vi "Autonomous Independent.vi"() -> ()   [LabVIEW 2020]
doc: "This VI is called when autonomous begins, and will automatically be terminated when autonomous ends. You can carry out timed or sensor driven robot movement independently without needing to return to the caller."
uses:
  <vilib>/Rock Robotics/WPI/Utilities/WPI_GetSetVariantRefNum.vi
  <vilib>/Rock Robotics/Network Tables/NT Read String.vi
  <vilib>/Rock Robotics/Network Tables/NT Write Numeric Array.vi
  <vilib>/Rock Robotics/Network Tables/NT Read Number.vi
  Robot Global Data.vi
  SUB VIs/TOGGLE GLOBAL.vi
  <vilib>/addons/control/pid/pid.llb/PID (DBL).vi
  ENUM_01.ctl
  <vilib>/addons/control/pid/NI_PID_pid.lvlib
panel:
  in  "CONTROL FREIO A3 2":dbl=-12.6
  in  "ACELERA敲O 3 A3 2":dbl=0.15
  in  "ACELERA敲O\n 3 A3 4":dbl=0.3
  in  "DISTANCE\nVOLTAR":dbl=1.6
  in  "TIMER 3 A3 2":dbl=500.0
  in  "ACELERA敲O 2 A3 2":dbl=-0.35
  in  "DISTANCIA A\nPERCORRER 2 A3 2":dbl=-4.0
  in  "TIMER 2 A3 2":dbl=50.0
  in  "DISTANCIA A\nPERCORRER 1 A3 2":dbl=0.1
  in  "ACELERA敲O 1 A3 2":dbl=0.3
  in  "TIMER 1 A3 2":dbl=150.0
  # "Be sure to right-click and choose Data Operations>>Make Current Value default if you want to save the array values with the VI"
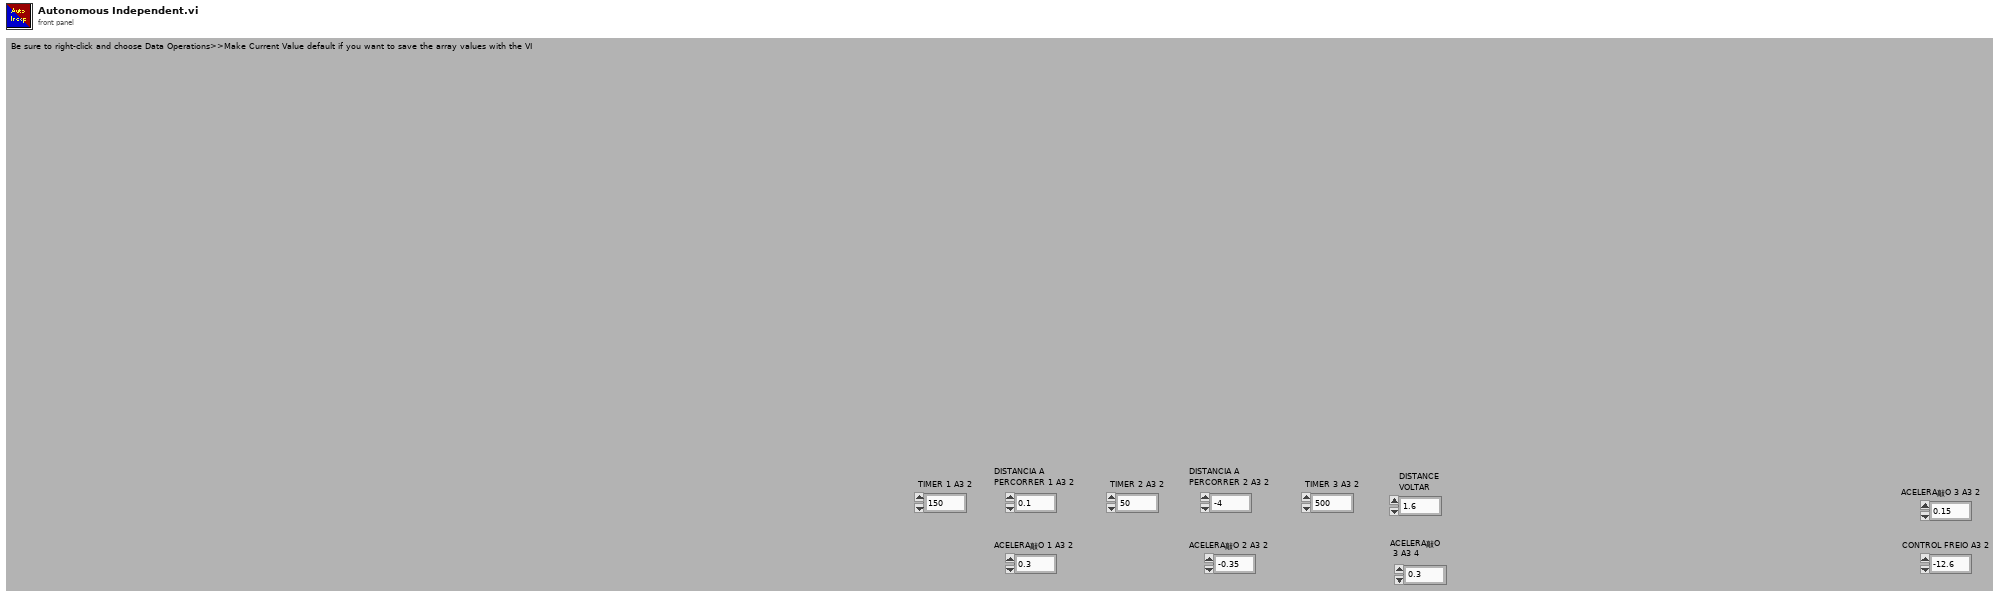
[diagram p1: front panel]
types:
  T1 = typedef "WPI_JoystickDevRef.ctl" = cluster{"Device":T2}
  T2 = typedef "WPI_JoystickDeviceEnum.ctl" = enum16{"USB 0", "USB 1", "USB 2", "USB 3", "USB 4", "USB 5"}
  T3 = enum16{"I00", "I01", "I02", "I03", "I04", "I05", "I06", "I07", "I08", "I09", "I10", "I11", "I12", "I13", "I14", "I15", "I16", "I17", "I18", "I19", "I20"}
  T4 = enum16{"I00", "I01", "I02", "I03", "I04", "I05", "I06", "I07", "I08", "I09", "I10", "I11", "I12", "I13", "I14", "I15"}
  T5 = cluster{"proportional gain (Kc)":dbl, "integral time (Ti, min)":dbl, "derivative time (Td, min)":dbl}
  T6 = typedef "ENUM_01.ctl" = enum16{"INICIO", "ANDA PARA FRENTE", "ESPERA 1", "ANDA PARA TRAS", "ESPERA 2", "VOLTA PARA A RAMPA", "INICIO EQUILIBRAR", "ESTABILIZA EQUILIBRIO", "FREIO", "ESPERA 3", "EQUILIBRIO"}
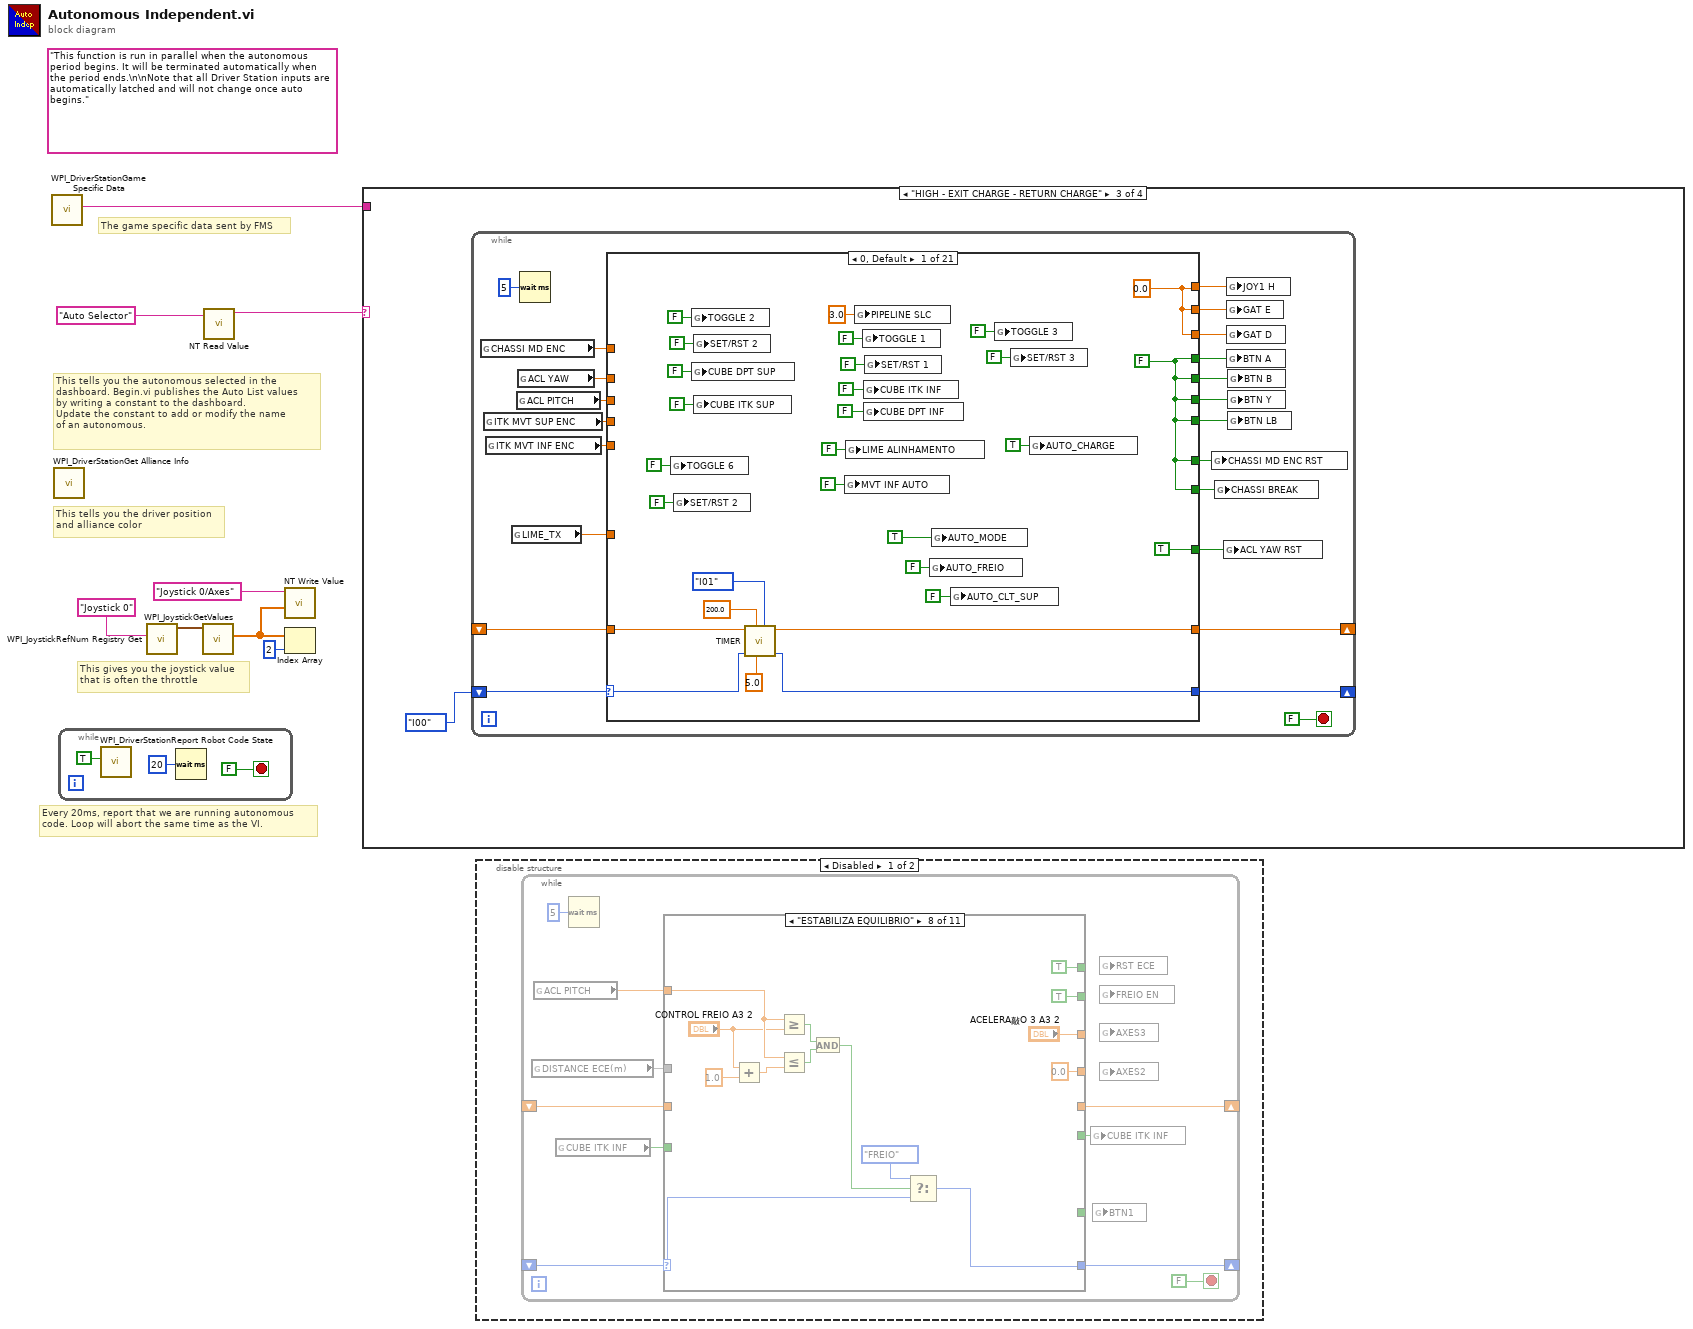
[diagram p0: block diagram]
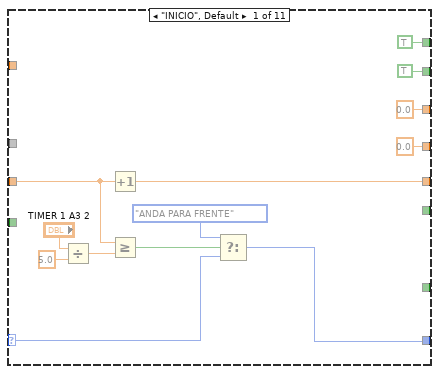
[diagram p2: hidden frame]
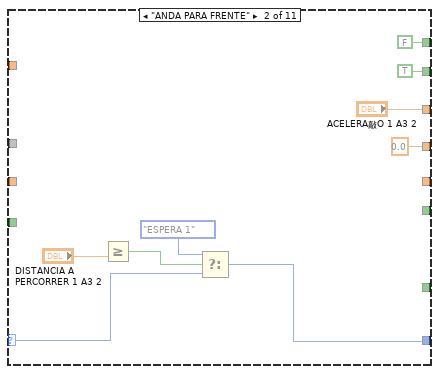
[diagram p3: hidden frame]
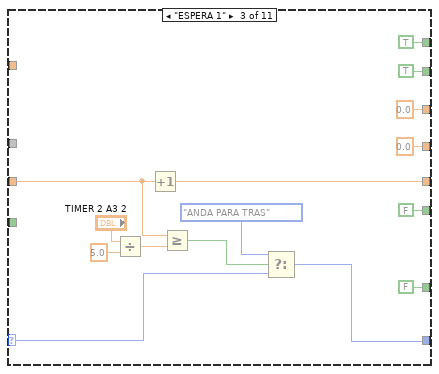
[diagram p4: hidden frame]
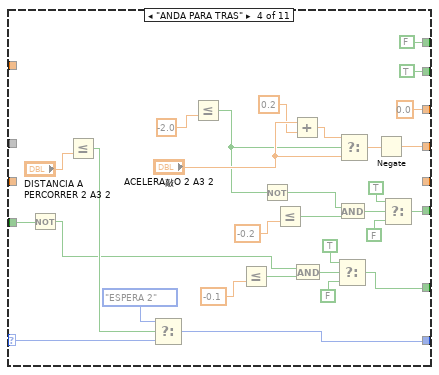
[diagram p5: hidden frame]
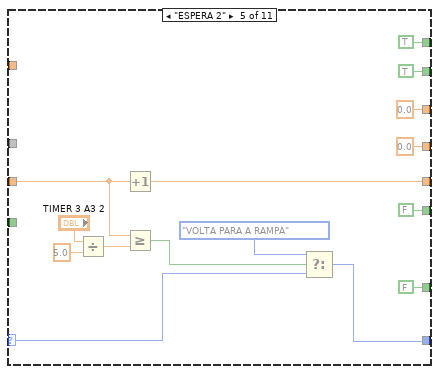
[diagram p6: hidden frame]
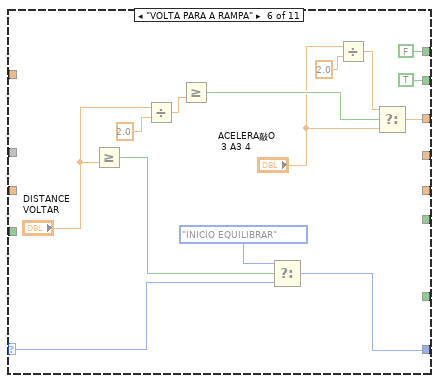
[diagram p7: hidden frame]
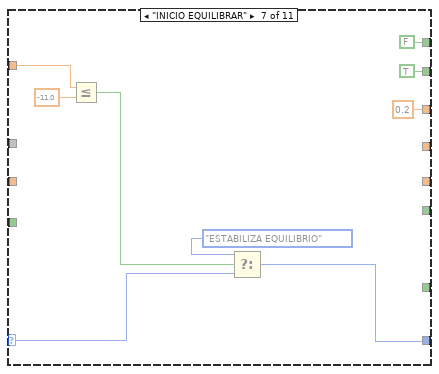
[diagram p8: hidden frame]
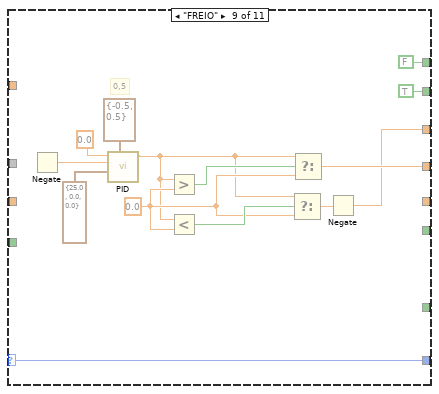
[diagram p9: hidden frame]
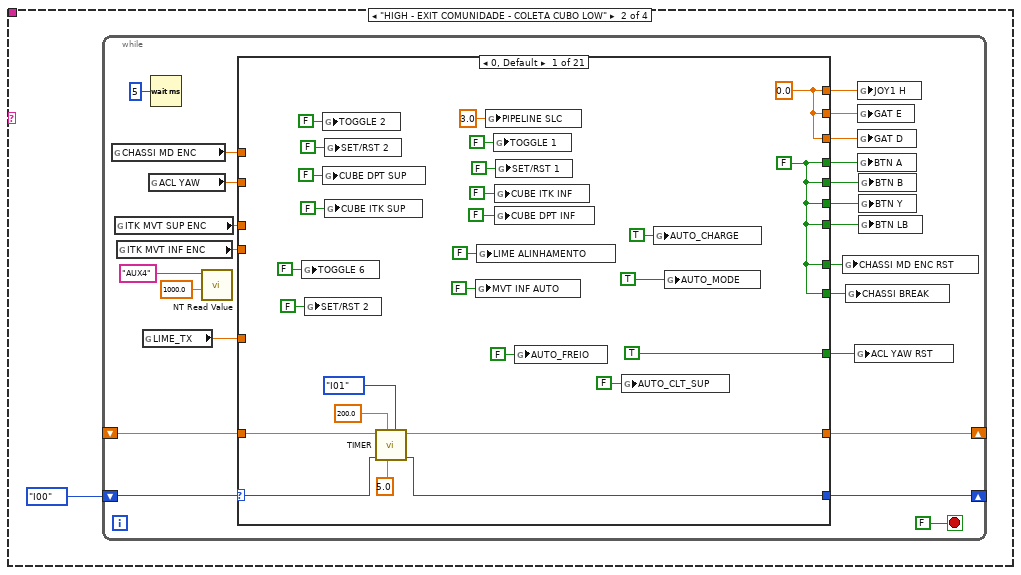
[diagram p14: hidden frame]
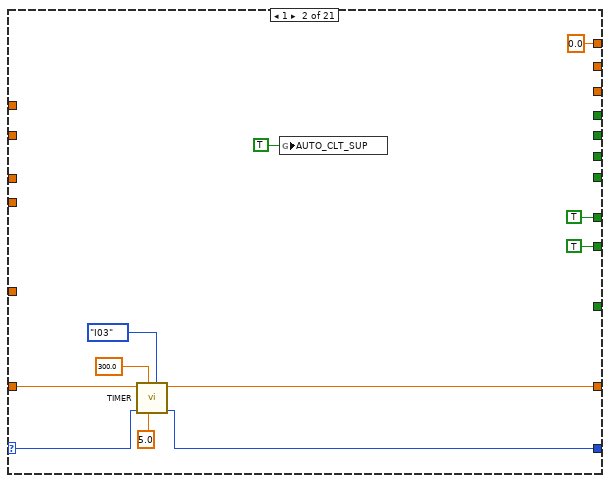
[diagram p15: hidden frame]
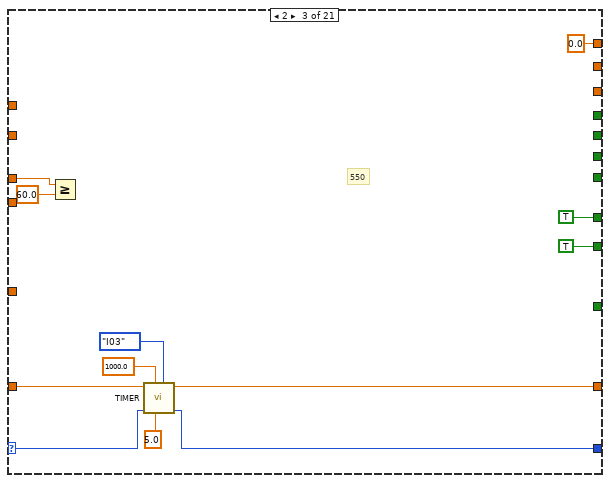
[diagram p16: hidden frame]
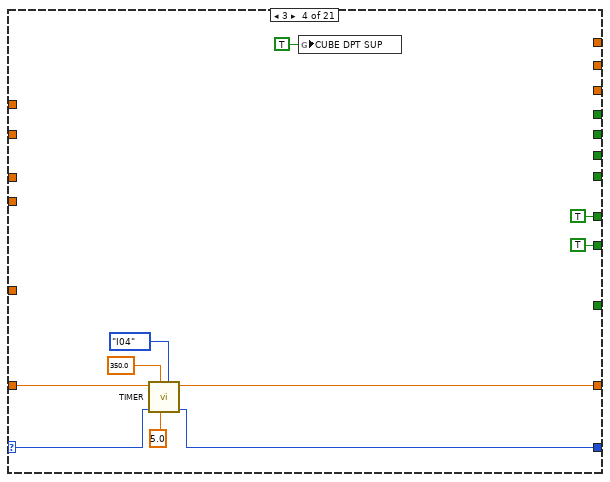
[diagram p17: hidden frame]
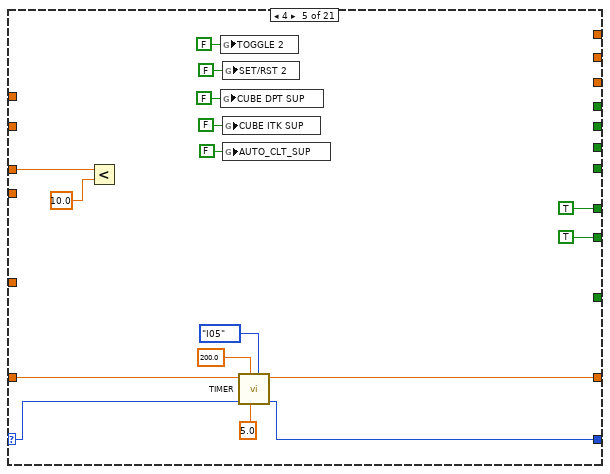
[diagram p18: hidden frame]
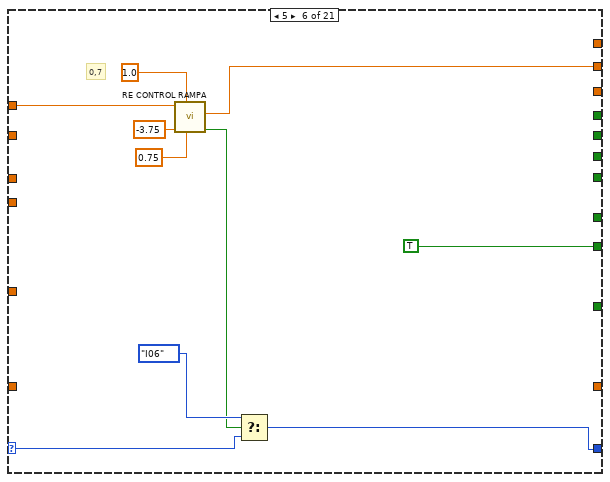
[diagram p19: hidden frame]
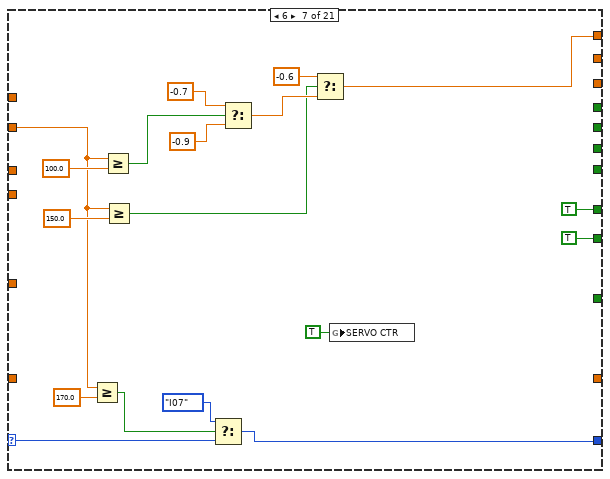
[diagram p20: hidden frame]
diagram:
  (unwired) "This function is run in parallel when the autonomous period begins. It will be terminated automatically when the period ends.\n\nNote that all Driver Station inputs are automatically latched and will not change once auto begins."
  # "The game specific data sent by FMS"
  # "This tells you the autonomous selected in the \ndashboard. Begin.vi publishes the Auto List values\nby writing a constant to the dashboard.\nUpdate the constant to add or modify the name\nof an autonomous."
  # "Every 20ms, report that we are running autonomous\ncode. Loop will abort the same time as the VI."
  # "This gives you the joystick value\nthat is often the throttle"
  # "This tells you the driver position\nand alliance color"
  n1 = call <vilib>:"WPI_DriverStationGame Specific Data.vi"() -> ("Game Specific Data"=w1:string)  [unwired: 11 in]
  n2 = call <vilib>:"WPI_DriverStationGet Alliance Info.vi"() -> ()  [unwired: 12 out]
  n3 = while {
    stop <- FALSE stop-if-true
    n4 = call <vilib>:"WPI_DriverStationReport Robot Code State.vi"("Autonomous"=TRUE) -> ()  [unwired: 10 in, 1 out]
    n5 = Wait (ms)(milliseconds to wait=u32 20) -> ()  [unwired: 1 out]
  }
  n6 = call <vilib>:"WPI_JoystickRefNum Registry Get.vi"("refnum name"="Joystick 0") -> ("JoystickDevRef"=w7:T1)  [unwired: 1 in, 9 out]
  n7 = call <vilib>:"WPI_JoystickGetValues.vi"("JoystickDevRef"=w7) -> ("Axes"=w3:dbl[])  [unwired: 6 in, 4 out]
  n8 = call-poly <vilib>:"NT Read Value.vi"("name"="Auto Selector" ("Name")) -> ("value"=w4:string)  [unwired: 8 in, 2 out]
  n9 = call-poly <vilib>:"NT Write Value.vi"("value"=w3, "name"="Joystick 0/Axes" ("Name")) -> ()  [unwired: 9 in, 1 out]
  n10 = Index Array(array=w3, index=2) -> ()  [unwired: 1 out]
  n11 = case shown="\"HIGH - EXIT CHARGE - RETURN CHARGE\"" w4 {
    tunnel: w1 -> [_ _ _ _]
    frame Default {
    }
    frame "HIGH - EXIT COMUNIDADE - COLETA CUBO LOW" {
      n12 = while {
        shift-right: [w35] -> _
        shift-left: _ -> [w34]
        shift-right: [w19] -> _
        shift-left: T3."I00" -> [w16]
        stop <- FALSE stop-if-true
        n13 = global read "Robot Global Data.vi" "CHASSI MD ENC"() -> (w24:dbl)
        n14 = global read "Robot Global Data.vi" "ITK MVT SUP ENC"() -> (w15:dbl)
        n15 = global read "Robot Global Data.vi" "ITK MVT INF ENC"() -> (w14:dbl)
        n16 = global read "Robot Global Data.vi" "LIME_TX"() -> (w13:dbl)
        n17 = global read "Robot Global Data.vi" "ACL YAW"() -> (w17:dbl)
        n18 = Wait (ms)(milliseconds to wait=u32 5) -> ()  [unwired: 1 out]
        n19 = call-poly <vilib>:"NT Read Value.vi"("default value"=1000.0, "name"="AUX4") -> ()  [unwired: 7 in, 3 out]
        n20 = case shown="0, Default" w16 {
          selector: w16 -> [w60 w69 w76 w92 w96 w117 w137 w143 w169 w196 w207 w215 w222 w237 w256 w283 w291 w304 w312 w328 _]
          tunnel: [w61 w68 w75 w90 w99 w118 w138 w142 w165 w195 w206 w214 w223 w236 w255 w259 w292 w302 w311 w328 _] -> w19
          tunnel: w34 -> [w57 w70 w78 w93 w97 _ _ w145 w154 w193 w204 _ _ _ w253 w274 _ w300 _ _ _]
          tunnel: [w58 w71 w77 w91 w98 _ _ w144 w170 w194 w205 _ _ _ w254 w284 _ w301 _ _ _] -> w35
          tunnel: [w62 0.0 ("f") 0.0 ("f") _ _ _ w135 0.3 ("f") _ _ _ _ _ w233 -0.3 ("f") _ _ _ w309 _ _] -> w31
          tunnel: [w62 _ _ _ _ w115 _ _ _ _ _ _ _ _ _ _ _ _ _ _ _] -> w30
          tunnel: [w62 _ _ _ _ _ _ _ _ _ _ _ w225 _ _ _ w293 _ _ _ _] -> w29
          tunnel: [w50 _ _ _ _ _ _ _ _ _ _ _ _ _ _ _ _ _ _ _ _] -> w28
          tunnel: [w50 _ _ _ _ _ _ _ _ _ _ _ _ _ _ _ _ _ _ _ _] -> w27
          tunnel: [w50 _ _ _ _ _ _ _ _ _ _ _ _ _ _ _ _ _ _ _ _] -> w26
          tunnel: [w50 _ _ _ _ _ _ _ _ _ _ _ _ _ _ _ _ _ _ _ _] -> w25
          tunnel: w24 -> [_ _ _ _ _ w116 _ _ _ _ _ _ w226 _ _ _ w294 _ _ _ _]
          tunnel: [w50 TRUE TRUE TRUE TRUE _ TRUE TRUE TRUE TRUE TRUE _ _ _ TRUE TRUE _ _ _ _ _] -> w23
          tunnel: [w50 TRUE TRUE TRUE TRUE TRUE TRUE TRUE TRUE TRUE TRUE _ TRUE TRUE TRUE TRUE TRUE TRUE _ _ _] -> w22
          tunnel: [TRUE _ _ _ _ _ _ _ _ _ _ _ _ _ _ _ _ _ _ _ _] -> w18
          tunnel: w17 -> [_ _ _ _ _ _ w125 _ _ _ _ _ _ w234 _ _ _ _ w310 _ _]
          tunnel: w15 -> [_ _ w83 _ w105 _ _ _ _ _ _ _ _ _ _ _ _ _ _ _ _]
          tunnel: w14 -> [_ _ _ _ _ _ _ _ _ _ _ w213 _ _ _ _ _ _ _ _ _]
          tunnel: w13 -> [_ _ _ _ _ _ _ _ _ _ _ _ _ _ _ _ _ _ _ _ _]
          frame 0, Default {
            w50 = FALSE
            w62 = 0.0 ("x")
            n21 = global write "TOGGLE GLOBAL.vi" "TOGGLE 6"(FALSE ("TOGGLE 6")) -> ()
            n22 = global write "TOGGLE GLOBAL.vi" "SET/RST 2"(FALSE ("SET/RST 2")) -> ()
            n23 = global write "TOGGLE GLOBAL.vi" "TOGGLE 2"(FALSE ("TOGGLE 2")) -> ()
            n24 = global write "Robot Global Data.vi" "CUBE DPT SUP"(FALSE ("CUBE DPT SUP")) -> ()
            n25 = global write "TOGGLE GLOBAL.vi" "SET/RST 2"(FALSE ("SET/RST 2")) -> ()
            n26 = global write "Robot Global Data.vi" "CUBE ITK SUP"(FALSE ("CUBE ITK SUP")) -> ()
            n27 = call "TIMER.vi"("NEXT CASE"=T4."I01", "CLK BASE"=5.0, "TIMER"=200.0, "ATUAL CASE"=w60, "CONTADOR"=w57) -> ("REALIMENTA敲O CASE"=w61:u16, "REALIMENTA敲O TIMER"=w58:dbl)  [unwired: 5 in]
            n28 = global write "Robot Global Data.vi" "MVT INF AUTO"(FALSE ("MVT INF AUTO")) -> ()
            n29 = global write "Robot Global Data.vi" "LIME ALINHAMENTO"(FALSE ("LIME ALINHAMENTO")) -> ()
            n30 = global write "Robot Global Data.vi" "PIPELINE SLC"(3.0 ("PIPELINE SLC")) -> ()
            n31 = global write "TOGGLE GLOBAL.vi" "TOGGLE 1"(FALSE ("TOGGLE 2")) -> ()
            n32 = global write "Robot Global Data.vi" "CUBE ITK INF"(FALSE ("CUBE ITK SUP")) -> ()
            n33 = global write "Robot Global Data.vi" "CUBE DPT INF"(FALSE ("CUBE DPT SUP")) -> ()
            n34 = global write "TOGGLE GLOBAL.vi" "SET/RST 1"(FALSE ("SET/RST 2")) -> ()
            n35 = global write "Robot Global Data.vi" "AUTO_FREIO"(FALSE ("AUTO_FREIO")) -> ()
            n36 = global write "Robot Global Data.vi" "AUTO_CLT_SUP"(FALSE ("AUTO_CLT")) -> ()
            n37 = global write "Robot Global Data.vi" "AUTO_CHARGE"(TRUE ("AUTO_CHARGE")) -> ()
            n38 = global write "Robot Global Data.vi" "AUTO_MODE"(TRUE ("CHASSI MD ENC RST")) -> ()
          }
          frame 1 {
            n39 = call "TIMER.vi"("NEXT CASE"=T4."I03", "CLK BASE"=5.0, "TIMER"=300.0, "ATUAL CASE"=w69, "CONTADOR"=w70) -> ("REALIMENTA敲O CASE"=w68:u16, "REALIMENTA敲O TIMER"=w71:dbl)  [unwired: 5 in]
            n40 = global write "Robot Global Data.vi" "AUTO_CLT_SUP"(TRUE ("AUTO_CLT")) -> ()
          }
          frame 2 {
            # "550"
            n41 = Greater Or Equal?(x=w83, y=60.0) -> ()  [unwired: 1 out]
            n42 = call "TIMER.vi"("NEXT CASE"=T4."I03", "CLK BASE"=5.0, "TIMER"=1000.0, "ATUAL CASE"=w76, "CONTADOR"=w78) -> ("REALIMENTA敲O CASE"=w75:u16, "REALIMENTA敲O TIMER"=w77:dbl)  [unwired: 5 in]
          }
          frame 3 {
            n43 = call "TIMER.vi"("NEXT CASE"=T4."I04", "CLK BASE"=5.0, "TIMER"=350.0, "ATUAL CASE"=w92, "CONTADOR"=w93) -> ("REALIMENTA敲O CASE"=w90:u16, "REALIMENTA敲O TIMER"=w91:dbl)  [unwired: 5 in]
            n44 = global write "Robot Global Data.vi" "CUBE DPT SUP"(TRUE ("CUBE DPT SUP")) -> ()
          }
          frame 4 {
            n45 = Less?(x=w105, y=10.0) -> ()  [unwired: 1 out]
            n46 = global write "TOGGLE GLOBAL.vi" "TOGGLE 2"(FALSE ("TOGGLE 2")) -> ()
            n47 = global write "Robot Global Data.vi" "CUBE DPT SUP"(FALSE ("CUBE DPT SUP")) -> ()
            n48 = global write "TOGGLE GLOBAL.vi" "SET/RST 2"(FALSE ("SET/RST 2")) -> ()
            n49 = global write "Robot Global Data.vi" "CUBE ITK SUP"(FALSE ("CUBE ITK SUP")) -> ()
            n50 = global write "Robot Global Data.vi" "AUTO_CLT_SUP"(FALSE ("AUTO_CLT")) -> ()
            n51 = call "TIMER.vi"("NEXT CASE"=T4."I05", "CLK BASE"=5.0, "TIMER"=200.0, "ATUAL CASE"=w96, "CONTADOR"=w97) -> ("REALIMENTA敲O CASE"=w99:u16, "REALIMENTA敲O TIMER"=w98:dbl)  [unwired: 5 in]
          }
          frame 5 {
            # "0,7"
            n52 = call "RE CONTROL RAMPA.vi"("RANGE SET POINT"=0.75, "V MAX"=1.0, "SET POINT"=-3.75, "DISTANCE IN"=w116) -> ("OK?"=w119:bool, "OUT RE"=w115:dbl)  [unwired: 6 in]
            n53 = Select(t=T4."I06", s=w119, f=w117) -> (s? t:f=w118:u16)
          }
          frame 6 {
            n54 = Greater Or Equal?(x=w125, y=170.0) -> (x >= y?=w133:bool)
            n55 = Greater Or Equal?(x=w125, y=100.0) -> (x >= y?=w127:bool)
            n56 = Greater Or Equal?(x=w125, y=150.0) -> (x >= y?=w124:bool)
            n57 = Select(t=T4."I07", s=w133, f=w137) -> (s? t:f=w138:u16)
            n58 = Select(t=-0.7 ("f"), s=w127, f=-0.9) -> (s? t:f=w131:dbl)
            n59 = Select(t=-0.6, s=w124, f=w131) -> (s? t:f=w135:dbl)
            n60 = global write "Robot Global Data.vi" "SERVO CTR"(TRUE ("SERVO CTR")) -> ()
          }
          frame 7 {
            n61 = call "TIMER.vi"("NEXT CASE"=T4."I08", "CLK BASE"=5.0, "TIMER"=100.0, "ATUAL CASE"=w143, "CONTADOR"=w145) -> ("REALIMENTA敲O CASE"=w142:u16, "REALIMENTA敲O TIMER"=w144:dbl)  [unwired: 5 in]
          }
          frame 8 {
            n62 = In Range and Coerce(upper limit=1000.0, x=w154, lower limit=801.0 ("y")) -> (In Range?=w156:bool)  [unwired: 1 out]
            n63 = In Range and Coerce(upper limit=400.0, x=w154, lower limit=301.0) -> (In Range?=w177:bool)  [unwired: 1 out]
            n64 = In Range and Coerce(upper limit=800.0, x=w154, lower limit=701.0) -> (In Range?=w159:bool)  [unwired: 1 out]
            n65 = Less Or Equal?(x=w154, y=300.0) -> (x <= y?=w183:bool)
            n66 = In Range and Coerce(upper limit=700.0, x=w154, lower limit=401.0) -> (In Range?=w175:bool)  [unwired: 1 out]
            n67 = Select(t=TRUE ("LIME ALINHAMENTO"), s=w183, f=FALSE) -> (s? t:f=w174:bool)
            n68 = call "TIMER.vi"("NEXT CASE"=T3."I09", "CLK BASE"=5.0, "TIMER"=1500.0, "ATUAL CASE"=w169, "CONTADOR"=w154) -> ("REALIMENTA敲O CASE"=w165:u16, "REALIMENTA敲O TIMER"=w170:dbl)  [unwired: 5 in]
            n69 = Select(t=FALSE ("LIME ALINHAMENTO"), s=w177, f=w174) -> (s? t:f=w173:bool)
            n70 = Select(t=TRUE ("LIME ALINHAMENTO"), s=w175, f=w173) -> (s? t:f=w171:bool)
            n71 = Greater Or Equal?(x=w154, y=1001.0) -> (x >= y?=w153:bool)
            n72 = Select(t=FALSE ("LIME ALINHAMENTO"), s=w159, f=w171) -> (s? t:f=w163:bool)
            n73 = Select(t=TRUE ("LIME ALINHAMENTO"), s=w156, f=w163) -> (s? t:f=w152:bool)
            n74 = Select(t=FALSE, s=w153, f=w152) -> (s? t:f=w150:bool)
            n75 = global write "Robot Global Data.vi" "LIME ALINHAMENTO"(w150) -> ()
          }
          frame 9 {
            n76 = call "TIMER.vi"("NEXT CASE"=T4."I10", "CLK BASE"=5.0, "TIMER"=100.0, "ATUAL CASE"=w196, "CONTADOR"=w193) -> ("REALIMENTA敲O CASE"=w195:u16, "REALIMENTA敲O TIMER"=w194:dbl)  [unwired: 5 in]
            n77 = global write "TOGGLE GLOBAL.vi" "TOGGLE 1"(FALSE ("TOGGLE 2")) -> ()
            n78 = global write "TOGGLE GLOBAL.vi" "SET/RST 1"(FALSE ("SET/RST 2")) -> ()
            n79 = global write "Robot Global Data.vi" "CUBE ITK INF"(FALSE ("CUBE DPT SUP")) -> ()
            n80 = global write "Robot Global Data.vi" "LIME ALINHAMENTO"(FALSE ("LIME ALINHAMENTO")) -> ()
          }
          frame 10 {
            (unwired) TRUE
            n81 = call "TIMER.vi"("NEXT CASE"=T4."I11", "CLK BASE"=5.0, "TIMER"=200.0, "ATUAL CASE"=w207, "CONTADOR"=w204) -> ("REALIMENTA敲O CASE"=w206:u16, "REALIMENTA敲O TIMER"=w205:dbl)  [unwired: 5 in]
            n82 = global write "Robot Global Data.vi" "MVT INF AUTO"(TRUE ("TOGGLE 1")) -> ()
          }
          frame 11 {
            n83 = Greater?(x=w213, y=50.0) -> (0:w211:bool)
            n84 = Select(t=T4."I12", s=w211, f=w215) -> (s? t:f=w214:u16)
          }
          frame 12 {
            n85 = call "FRENTE CONTROL RAMPA.vi"("RANGE SET POINT"=0.35, "V MAX"=0.85, "SET POINT"=0.5, "DISTANCE IN"=w226) -> ("OK?"=w220:bool, "OUT FRENTE"=w225:dbl)  [unwired: 5 in, 1 out]
            n86 = Select(t=T4."I13", s=w220, f=w222) -> (s? t:f=w223:u16)
          }
          frame 13 {
            n87 = Less Or Equal?(x=w234, y=20.0) -> (x <= y?=w232:bool)
            n88 = Less Or Equal?(x=w234, y=80.0) -> (x <= y?=w229:bool)
            n89 = Less Or Equal?(x=w234, y=30.0) -> (x <= y?=w227:bool)
            n90 = global read "Robot Global Data.vi" "CUBE ITK INF"() -> (w231:bool)
            n91 = Select(t=0.7 ("f"), s=w229, f=0.9) -> (s? t:f=w243:dbl)
            n92 = Select(t=T3."I14", s=w232, f=w237) -> (s? t:f=w236:u16)
            n93 = Select(t=0.6, s=w227, f=w243) -> (s? t:f=w233:dbl)
            n94 = Not(x=w231) -> (.not. x?=w230:bool)
            n95 = global write "Robot Global Data.vi" "SERVO CTR"(TRUE ("SERVO CTR")) -> ()
            n96 = And(x=w227, y=w230) -> (x .and. y?=w228:bool)
            n97 = case shown="True" w228 {
              frame False {
              }
              frame True {
                n98 = global write "Robot Global Data.vi" "MVT INF AUTO"(FALSE ("MVT INF AUTO")) -> ()
              }
            }
          }
          frame 14 {
            n99 = call "TIMER.vi"("NEXT CASE"=T3."I19", "CLK BASE"=5.0, "TIMER"=100.0, "ATUAL CASE"=w256, "CONTADOR"=w253) -> ("REALIMENTA敲O CASE"=w255:u16, "REALIMENTA敲O TIMER"=w254:dbl)  [unwired: 5 in]
            n100 = global write "Robot Global Data.vi" "SERVO CTR"(FALSE ("SERVO CTR")) -> ()
          }
          frame 15 {
            n101 = In Range and Coerce(upper limit=400.0, x=w274, lower limit=301.0) -> (In Range?=w272:bool)  [unwired: 1 out]
            n102 = Less Or Equal?(x=w274, y=300.0) -> (x <= y?=w280:bool)
            n103 = In Range and Coerce(upper limit=700.0, x=w274, lower limit=401.0) -> (In Range?=w270:bool)  [unwired: 1 out]
            n104 = Greater Or Equal?(x=w274, y=701.0) -> (x >= y?=w265:bool)
            n105 = Select(t=TRUE ("LIME ALINHAMENTO"), s=w280, f=FALSE) -> (s? t:f=w269:bool)
            n106 = call "TIMER.vi"("NEXT CASE"=T4."I09", "CLK BASE"=5.0, "TIMER"=800.0, "ATUAL CASE"=w283, "CONTADOR"=w274) -> ("REALIMENTA敲O CASE"=w259:u16, "REALIMENTA敲O TIMER"=w284:dbl)  [unwired: 5 in]
            n107 = Select(t=FALSE ("LIME ALINHAMENTO"), s=w272, f=w269) -> (s? t:f=w268:bool)
            n108 = Select(t=TRUE ("LIME ALINHAMENTO"), s=w270, f=w268) -> (s? t:f=w266:bool)
            n109 = Select(t=FALSE ("LIME ALINHAMENTO"), s=w265, f=w266) -> (s? t:f=w264:bool)
            n110 = global write "Robot Global Data.vi" "LIME ALINHAMENTO"(w264) -> ()
          }
          frame 16 {
            n111 = call "FRENTE CONTROL RAMPA.vi"("RANGE SET POINT"=0.4, "V MAX"=1.0, "SET POINT"=1.0, "DISTANCE IN"=w294) -> ("OK?"=w296:bool, "OUT FRENTE"=w293:dbl)  [unwired: 5 in, 1 out]
            n112 = global write "Robot Global Data.vi" "LIME ALINHAMENTO"(FALSE ("LIME ALINHAMENTO")) -> ()
            n113 = Select(t=T3."I17", s=w296, f=w291) -> (s? t:f=w292:u16)
          }
          frame 17 {
            n114 = call "TIMER.vi"("NEXT CASE"=T3."I18", "CLK BASE"=5.0, "TIMER"=200.0, "ATUAL CASE"=w304, "CONTADOR"=w300) -> ("REALIMENTA敲O CASE"=w302:u16, "REALIMENTA敲O TIMER"=w301:dbl)  [unwired: 5 in]
            n115 = global write "Robot Global Data.vi" "CUBE DPT INF"(TRUE ("CUBE DPT SUP")) -> ()
          }
          frame 18 {
            (unwired) TRUE
            (unwired) TRUE
            n116 = Greater Or Equal?(x=w310, y=80.0) -> (x >= y?=w322:bool)
            n117 = Greater Or Equal?(x=w310, y=40.0) -> (x >= y?=w316:bool)
            n118 = Greater Or Equal?(x=w310, y=60.0) -> (x >= y?=w314:bool)
            n119 = Select(t=T3."I19", s=w322, f=w312) -> (s? t:f=w311:u16)
            n120 = Select(t=-0.7 ("f"), s=w316, f=-0.9) -> (s? t:f=w320:dbl)
            n121 = global write "Robot Global Data.vi" "ITK INF AUTO"(FALSE ("ITK INF AUTO")) -> ()
            n122 = Select(t=-0.6, s=w314, f=w320) -> (s? t:f=w309:dbl)
            n123 = global write "Robot Global Data.vi" "SERVO CTR"(TRUE ("SERVO CTR")) -> ()
          }
          frame 19 {
            n124 = disable-structure shown="Disabled" {
              frame Disabled {
                n125 = global write "TOGGLE GLOBAL.vi" "TOGGLE 1"(FALSE ("TOGGLE 2")) -> ()
                n126 = global write "TOGGLE GLOBAL.vi" "SET/RST 1"(FALSE ("SET/RST 2")) -> ()
                n127 = global write "Robot Global Data.vi" "CUBE ITK INF"(FALSE ("CUBE DPT SUP")) -> ()
              }
              frame Enabled {
              }
            }
            n128 = global write "Robot Global Data.vi" "SERVO CTR"(FALSE ("SERVO CTR")) -> ()
            n129 = global write "Robot Global Data.vi" "CUBE ITK SUP"(FALSE ("CUBE ITK SUP")) -> ()
            n130 = global write "Robot Global Data.vi" "AUTO_MODE"(FALSE ("CHASSI MD ENC RST")) -> ()
            n131 = global write "Robot Global Data.vi" "MVT INF AUTO"(FALSE ("MVT INF AUTO")) -> ()
          }
          frame 20 {
          }
        }
        n132 = global write "Robot Global Data.vi" "CHASSI MD ENC RST"(w23) -> ()
        n133 = global write "Robot Global Data.vi" "CHASSI BREAK"(w22) -> ()
        n134 = global write "Robot Global Data.vi" "ACL YAW RST"(w18) -> ()
        n135 = global write "Robot Global Data.vi" "JOY1 H"(w31) -> ()
        n136 = global write "Robot Global Data.vi" "GAT E"(w30) -> ()
        n137 = global write "Robot Global Data.vi" "GAT D"(w29) -> ()
        n138 = global write "Robot Global Data.vi" "BTN A"(w28) -> ()
        n139 = global write "Robot Global Data.vi" "BTN B"(w27) -> ()
        n140 = global write "Robot Global Data.vi" "BTN Y"(w26) -> ()
        n141 = global write "Robot Global Data.vi" "BTN LB"(w25) -> ()
      }
    }
    frame "HIGH - EXIT CHARGE - RETURN CHARGE" {
      n142 = while {
        shift-right: [w354] -> _
        shift-left: _ -> [w353]
        shift-right: [w340] -> _
        shift-left: T3."I00" -> [w337]
        stop <- FALSE stop-if-true
        n143 = global read "Robot Global Data.vi" "CHASSI MD ENC"() -> (w343:dbl)
        n144 = global read "Robot Global Data.vi" "ITK MVT SUP ENC"() -> (w336:dbl)
        n145 = global read "Robot Global Data.vi" "ITK MVT INF ENC"() -> (w335:dbl)
        n146 = global read "Robot Global Data.vi" "LIME_TX"() -> (w334:dbl)
        n147 = global read "Robot Global Data.vi" "ACL PITCH"() -> (w333:dbl)
        n148 = global read "Robot Global Data.vi" "ACL YAW"() -> (w338:dbl)
        n149 = Wait (ms)(milliseconds to wait=u32 5) -> ()  [unwired: 1 out]
        n150 = case shown="0, Default" w337 {
          selector: w337 -> [w381 w390 w396 w420 w424 w445 w451 w470 w480 w486 _ w513 w520 w530 w550 w577 w585 w598 w606 w621 _]
          tunnel: [w382 w389 w397 w418 w427 w446 w453 w469 w479 w488 _ w513 w521 w529 w549 w553 w586 w596 w605 w621 _] -> w340
          tunnel: w353 -> [w378 w391 w405 w421 w425 _ w450 _ _ _ _ _ _ _ w547 w568 _ w594 _ _ _]
          tunnel: [w379 w392 w406 w419 w426 _ w452 _ _ _ _ _ _ _ w548 w578 _ w595 _ _ _] -> w354
          tunnel: [w383 _ _ _ _ _ _ _ _ _ _ _ _ w526 -0.3 ("f") _ _ _ w603 _ _] -> w350
          tunnel: [w383 _ _ _ _ w443 _ _ _ _ _ w502 _ _ _ _ _ _ _ _ _] -> w349
          tunnel: [w383 _ _ _ _ _ _ w461 _ 0.245 ("OUT FRENTE") _ w503 w523 _ _ _ w587 _ _ _ _] -> w348
          tunnel: [w371 _ _ _ _ _ _ _ _ _ _ _ _ _ _ _ _ _ _ _ _] -> w347
          tunnel: [w371 _ _ _ _ _ _ _ _ _ _ _ _ _ _ _ _ _ _ _ _] -> w346
          tunnel: [w371 TRUE _ _ _ _ _ _ _ _ _ _ _ _ _ _ _ _ _ _ _] -> w345
          tunnel: [w371 _ TRUE _ _ _ _ _ _ _ _ _ _ _ _ _ _ _ _ _ _] -> w344
          tunnel: w343 -> [_ _ _ _ _ w444 _ w467 _ _ _ w501 w524 _ _ _ w588 _ _ _ _]
          tunnel: [w371 TRUE TRUE TRUE TRUE _ TRUE _ TRUE TRUE _ _ _ _ TRUE TRUE _ _ _ _ _] -> w342
          tunnel: [w371 TRUE TRUE TRUE TRUE TRUE TRUE TRUE TRUE TRUE _ TRUE TRUE TRUE TRUE TRUE TRUE TRUE _ _ _] -> w341
          tunnel: [TRUE _ _ _ _ _ _ _ _ _ _ _ _ _ _ _ _ _ _ _ _] -> w339
          tunnel: w338 -> [_ _ _ _ _ _ _ _ _ _ _ _ _ w527 _ _ _ _ w604 _ _]
          tunnel: w336 -> [_ _ w400 _ w433 _ _ _ _ _ _ _ _ _ _ _ _ _ _ _ _]
          tunnel: w335 -> [_ _ _ _ _ _ _ _ _ _ _ _ _ _ _ _ _ _ _ _ _]
          tunnel: w334 -> [_ _ _ _ _ _ _ _ _ _ _ _ _ _ _ _ _ _ _ _ _]
          tunnel: w333 -> [_ _ _ _ _ _ _ _ w476 w489 _ _ _ _ _ _ _ _ _ _ _]
          frame 0, Default {
            w371 = FALSE
            w383 = 0.0 ("x")
            n151 = global write "TOGGLE GLOBAL.vi" "TOGGLE 6"(FALSE ("TOGGLE 6")) -> ()
            n152 = global write "TOGGLE GLOBAL.vi" "SET/RST 2"(FALSE ("SET/RST 2")) -> ()
            n153 = global write "TOGGLE GLOBAL.vi" "TOGGLE 2"(FALSE ("TOGGLE 2")) -> ()
            n154 = global write "Robot Global Data.vi" "CUBE DPT SUP"(FALSE ("CUBE DPT SUP")) -> ()
            n155 = global write "TOGGLE GLOBAL.vi" "SET/RST 2"(FALSE ("SET/RST 2")) -> ()
            n156 = global write "Robot Global Data.vi" "CUBE ITK SUP"(FALSE ("CUBE ITK SUP")) -> ()
            n157 = call "TIMER.vi"("NEXT CASE"=T4."I01", "CLK BASE"=5.0, "TIMER"=200.0, "ATUAL CASE"=w381, "CONTADOR"=w378) -> ("REALIMENTA敲O CASE"=w382:u16, "REALIMENTA敲O TIMER"=w379:dbl)  [unwired: 5 in]
            n158 = global write "Robot Global Data.vi" "MVT INF AUTO"(FALSE ("MVT INF AUTO")) -> ()
            n159 = global write "Robot Global Data.vi" "LIME ALINHAMENTO"(FALSE ("LIME ALINHAMENTO")) -> ()
            n160 = global write "Robot Global Data.vi" "PIPELINE SLC"(3.0 ("PIPELINE SLC")) -> ()
            n161 = global write "TOGGLE GLOBAL.vi" "TOGGLE 1"(FALSE ("TOGGLE 2")) -> ()
            n162 = global write "Robot Global Data.vi" "CUBE ITK INF"(FALSE ("CUBE ITK SUP")) -> ()
            n163 = global write "Robot Global Data.vi" "CUBE DPT INF"(FALSE ("CUBE DPT SUP")) -> ()
            n164 = global write "TOGGLE GLOBAL.vi" "SET/RST 1"(FALSE ("SET/RST 2")) -> ()
            n165 = global write "Robot Global Data.vi" "AUTO_FREIO"(FALSE ("AUTO_FREIO")) -> ()
            n166 = global write "Robot Global Data.vi" "AUTO_MODE"(TRUE ("CHASSI MD ENC RST")) -> ()
            n167 = global write "Robot Global Data.vi" "AUTO_CLT_SUP"(FALSE ("AUTO_CLT")) -> ()
            n168 = global write "TOGGLE GLOBAL.vi" "TOGGLE 3"(FALSE ("TOGGLE 3")) -> ()
            n169 = global write "TOGGLE GLOBAL.vi" "SET/RST 3"(FALSE ("SET/RST 2")) -> ()
            n170 = global write "Robot Global Data.vi" "AUTO_CHARGE"(TRUE ("AUTO_CHARGE")) -> ()
          }
          frame 1 {
            n171 = call "TIMER.vi"("NEXT CASE"=T4."I03", "CLK BASE"=5.0, "TIMER"=300.0, "ATUAL CASE"=w390, "CONTADOR"=w391) -> ("REALIMENTA敲O CASE"=w389:u16, "REALIMENTA敲O TIMER"=w392:dbl)  [unwired: 5 in]
            n172 = global write "Robot Global Data.vi" "AUTO_CLT_SUP"(TRUE ("AUTO_CLT")) -> ()
          }
          frame 2 {
            n173 = Greater Or Equal?(x=w400, y=60.0) -> (x >= y?=w395:bool)
            n174 = disable-structure shown="Disabled" {
              disable-tunnel: [w412 _] -> w406
              disable-tunnel: [w411 _] -> _
              disable-tunnel: w396 -> [w410 _]
              disable-tunnel: w405 -> [w409 _]
              frame Disabled {
                # "550"
                n175 = call "TIMER.vi"("NEXT CASE"=T4."I03", "CLK BASE"=5.0, "TIMER"=1000.0, "ATUAL CASE"=w410, "CONTADOR"=w409) -> ("REALIMENTA敲O CASE"=w411:u16, "REALIMENTA敲O TIMER"=w412:dbl)  [unwired: 5 in]
              }
              frame Enabled {
              }
            }
            n176 = global write "Robot Global Data.vi" "CUBE DPT SUP"(FALSE ("CUBE DPT SUP")) -> ()
            n177 = Select(t=T4."I03", s=w395, f=w396) -> (s? t:f=w397:u16)
          }
          frame 3 {
            n178 = call "TIMER.vi"("NEXT CASE"=T4."I04", "CLK BASE"=5.0, "TIMER"=350.0, "ATUAL CASE"=w420, "CONTADOR"=w421) -> ("REALIMENTA敲O CASE"=w418:u16, "REALIMENTA敲O TIMER"=w419:dbl)  [unwired: 5 in]
            n179 = global write "Robot Global Data.vi" "CUBE DPT SUP"(TRUE ("CUBE DPT SUP")) -> ()
          }
          frame 4 {
            n180 = Less?(x=w433, y=10.0) -> ()  [unwired: 1 out]
            n181 = global write "Robot Global Data.vi" "AUTO_CLT_SUP"(FALSE ("AUTO_CLT")) -> ()
            n182 = global write "TOGGLE GLOBAL.vi" "TOGGLE 2"(FALSE ("TOGGLE 2")) -> ()
            n183 = global write "Robot Global Data.vi" "CUBE DPT SUP"(FALSE ("CUBE DPT SUP")) -> ()
            n184 = global write "TOGGLE GLOBAL.vi" "SET/RST 2"(FALSE ("SET/RST 2")) -> ()
            n185 = global write "Robot Global Data.vi" "CUBE ITK SUP"(FALSE ("CUBE ITK SUP")) -> ()
            n186 = call "TIMER.vi"("NEXT CASE"=T4."I05", "CLK BASE"=5.0, "TIMER"=200.0, "ATUAL CASE"=w424, "CONTADOR"=w425) -> ("REALIMENTA敲O CASE"=w427:u16, "REALIMENTA敲O TIMER"=w426:dbl)  [unwired: 5 in]
          }
          frame 5 {
            # "0,7"
            n187 = call "RE CONTROL RAMPA.vi"("RANGE SET POINT"=1.0, "V MAX"=0.6, "SET POINT"=-3.4, "DISTANCE IN"=w444) -> ("OK?"=w447:bool, "OUT RE"=w443:dbl)  [unwired: 6 in]
            n188 = Select(t=T4."I06", s=w447, f=w445) -> (s? t:f=w446:u16)
          }
          frame 6 {
            n189 = call "TIMER.vi"("NEXT CASE"=T4."I07", "CLK BASE"=5.0, "TIMER"=1000.0, "ATUAL CASE"=w451, "CONTADOR"=w450) -> ("REALIMENTA敲O CASE"=w453:u16, "REALIMENTA敲O TIMER"=w452:dbl)  [unwired: 5 in]
          }
          frame 7 {
            n190 = call "FRENTE CONTROL RAMPA.vi"("RANGE SET POINT"=1.0, "V MAX"=0.85, "SET POINT"=1.6, "DISTANCE IN"=w467) -> ("OK?"=w468:bool, "OUT FRENTE"=w464:dbl, "1STG?"=w460:bool)  [unwired: 5 in]
            n191 = global write "Robot Global Data.vi" "AUTO_CHARGE"(FALSE ("AUTO_CHARGE")) -> ()
            n192 = Select(t=T4."I09", s=w468, f=w470) -> (s? t:f=w469:u16)
            n193 = Select(t=0.2, s=w460, f=0.0) -> (s? t:f=w463:dbl)
            n194 = Add(x=w463, y=w464) -> (x+y=w462:dbl)
            n195 = Select(t=w462, s=w460, f=w464) -> (s? t:f=w461:dbl)
          }
          frame 8 {
            n196 = Less Or Equal?(x=w476, y=-12.5) -> (x <= y?=w477:bool)
            n197 = Select(t=T3."I09", s=w477, f=w480) -> (s? t:f=w479:u16)
          }
          frame 9 {
            w484 = -9.4 ("y")
            n198 = Add(x=w484, y=1.0) -> (x+y=w491:dbl)
            n199 = Greater Or Equal?(x=w489, y=w484) -> (x >= y?=w493:bool)
            n200 = Less Or Equal?(x=w489, y=w491) -> (x <= y?=w492:bool)
            n201 = And(x=w493, y=w492) -> (x .and. y?=w485:bool)
            n202 = Select(t=T4."I11", s=w485, f=w486) -> (s? t:f=w488:u16)
          }
          frame 10 {
            (unwired) T4."I11"
          }
          frame 11 {
            w507 = 0.0 ("y")
            (unwired) T4."I11"
            n203 = Negate(x=w501) -> (-x=w504:dbl)
            n204 = call-poly <vilib>:"PID.vi"("output range"=cluster{"output high":dbl, "output low":dbl} {"output high"=-0.5, "output low"=0.5}, "PID gains"=T5 {"proportional gain (Kc)"=25.0, "integral time (Ti, min)"=0.0, "derivative time (Td, min)"=0.0}, "process variable"=w504, "setpoint"=0.0) -> ("output"=w505:dbl)  [unwired: 6 in, 1 out]
            n205 = Greater?(x=w505, y=w507) -> (0:w509:bool)
            n206 = Less?(x=w505, y=w507) -> (x < y?=w508:bool)
            n207 = global write "Robot Global Data.vi" "LIME ALINHAMENTO"(FALSE ("LIME ALINHAMENTO")) -> ()
            n208 = global write "TOGGLE GLOBAL.vi" "TOGGLE 1"(FALSE ("TOGGLE 2")) -> ()
            n209 = global write "TOGGLE GLOBAL.vi" "SET/RST 1"(FALSE ("SET/RST 2")) -> ()
            n210 = global write "Robot Global Data.vi" "CUBE ITK INF"(FALSE ("CUBE DPT SUP")) -> ()
            n211 = Select(t=w505, s=w508, f=w507) -> (s? t:f=w506:dbl)
            n212 = Select(t=w505, s=w509, f=w507) -> (s? t:f=w502:dbl)
            n213 = Negate(x=w506) -> (-x=w503:dbl)
          }
          frame 12 {
            n214 = call "FRENTE CONTROL RAMPA.vi"("RANGE SET POINT"=0.35, "V MAX"=0.85, "SET POINT"=0.5, "DISTANCE IN"=w524) -> ("OK?"=w518:bool, "OUT FRENTE"=w523:dbl)  [unwired: 5 in, 1 out]
            n215 = Select(t=T4."I13", s=w518, f=w520) -> (s? t:f=w521:u16)
          }
          frame 13 {
            n216 = Less Or Equal?(x=w527, y=20.0) -> (x <= y?=w525:bool)
            n217 = Less Or Equal?(x=w527, y=80.0) -> (x <= y?=w534:bool)
            n218 = Less Or Equal?(x=w527, y=30.0) -> (x <= y?=w532:bool)
            n219 = Select(t=0.23 ("f"), s=w534, f=0.3) -> (s? t:f=w538:dbl)
            n220 = Select(t=T3."I14", s=w525, f=w530) -> (s? t:f=w529:u16)
            n221 = Select(t=0.15, s=w532, f=w538) -> (s? t:f=w526:dbl)
            n222 = global write "Robot Global Data.vi" "SERVO CTR"(TRUE ("SERVO CTR")) -> ()
          }
          frame 14 {
            n223 = call "TIMER.vi"("NEXT CASE"=T3."I19", "CLK BASE"=5.0, "TIMER"=100.0, "ATUAL CASE"=w550, "CONTADOR"=w547) -> ("REALIMENTA敲O CASE"=w549:u16, "REALIMENTA敲O TIMER"=w548:dbl)  [unwired: 5 in]
            n224 = global write "Robot Global Data.vi" "SERVO CTR"(FALSE ("SERVO CTR")) -> ()
          }
          frame 15 {
            n225 = In Range and Coerce(upper limit=400.0, x=w568, lower limit=301.0) -> (In Range?=w566:bool)  [unwired: 1 out]
            n226 = Less Or Equal?(x=w568, y=300.0) -> (x <= y?=w574:bool)
            n227 = In Range and Coerce(upper limit=700.0, x=w568, lower limit=401.0) -> (In Range?=w564:bool)  [unwired: 1 out]
            n228 = Greater Or Equal?(x=w568, y=701.0) -> (x >= y?=w559:bool)
            n229 = Select(t=TRUE ("LIME ALINHAMENTO"), s=w574, f=FALSE) -> (s? t:f=w563:bool)
            n230 = call "TIMER.vi"("NEXT CASE"=T4."I09", "CLK BASE"=5.0, "TIMER"=800.0, "ATUAL CASE"=w577, "CONTADOR"=w568) -> ("REALIMENTA敲O CASE"=w553:u16, "REALIMENTA敲O TIMER"=w578:dbl)  [unwired: 5 in]
            n231 = Select(t=FALSE ("LIME ALINHAMENTO"), s=w566, f=w563) -> (s? t:f=w562:bool)
            n232 = Select(t=TRUE ("LIME ALINHAMENTO"), s=w564, f=w562) -> (s? t:f=w560:bool)
            n233 = Select(t=FALSE ("LIME ALINHAMENTO"), s=w559, f=w560) -> (s? t:f=w558:bool)
            n234 = global write "Robot Global Data.vi" "LIME ALINHAMENTO"(w558) -> ()
          }
          frame 16 {
            n235 = call "FRENTE CONTROL RAMPA.vi"("RANGE SET POINT"=0.35, "V MAX"=1.0, "SET POINT"=1.0, "DISTANCE IN"=w588) -> ("OK?"=w590:bool, "OUT FRENTE"=w587:dbl)  [unwired: 5 in, 1 out]
            n236 = global write "Robot Global Data.vi" "LIME ALINHAMENTO"(FALSE ("LIME ALINHAMENTO")) -> ()
            n237 = Select(t=T3."I17", s=w590, f=w585) -> (s? t:f=w586:u16)
          }
          frame 17 {
            n238 = call "TIMER.vi"("NEXT CASE"=T3."I18", "CLK BASE"=5.0, "TIMER"=200.0, "ATUAL CASE"=w598, "CONTADOR"=w594) -> ("REALIMENTA敲O CASE"=w596:u16, "REALIMENTA敲O TIMER"=w595:dbl)  [unwired: 5 in]
            n239 = global write "Robot Global Data.vi" "CUBE DPT INF"(TRUE ("CUBE DPT SUP")) -> ()
          }
          frame 18 {
            (unwired) TRUE
            (unwired) TRUE
            n240 = Greater Or Equal?(x=w604, y=80.0) -> (x >= y?=w616:bool)
            n241 = Greater Or Equal?(x=w604, y=40.0) -> (x >= y?=w610:bool)
            n242 = Greater Or Equal?(x=w604, y=60.0) -> (x >= y?=w608:bool)
            n243 = Select(t=T3."I19", s=w616, f=w606) -> (s? t:f=w605:u16)
            n244 = Select(t=-0.3 ("f"), s=w610, f=-0.36) -> (s? t:f=w614:dbl)
            n245 = global write "Robot Global Data.vi" "ITK INF AUTO"(FALSE ("ITK INF AUTO")) -> ()
            n246 = Select(t=-0.25, s=w608, f=w614) -> (s? t:f=w603:dbl)
            n247 = global write "Robot Global Data.vi" "SERVO CTR"(TRUE ("SERVO CTR")) -> ()
          }
          frame 19 {
            n248 = disable-structure shown="Disabled" {
              frame Disabled {
                n249 = global write "TOGGLE GLOBAL.vi" "TOGGLE 1"(FALSE ("TOGGLE 2")) -> ()
                n250 = global write "TOGGLE GLOBAL.vi" "SET/RST 1"(FALSE ("SET/RST 2")) -> ()
                n251 = global write "Robot Global Data.vi" "CUBE ITK INF"(FALSE ("CUBE DPT SUP")) -> ()
              }
              frame Enabled {
              }
            }
            n252 = global write "Robot Global Data.vi" "SERVO CTR"(FALSE ("SERVO CTR")) -> ()
            n253 = global write "Robot Global Data.vi" "CUBE ITK SUP"(FALSE ("CUBE ITK SUP")) -> ()
            n254 = global write "Robot Global Data.vi" "MVT INF AUTO"(FALSE ("MVT INF AUTO")) -> ()
          }
          frame 20 {
          }
        }
        n255 = global write "Robot Global Data.vi" "CHASSI MD ENC RST"(w342) -> ()
        n256 = global write "Robot Global Data.vi" "CHASSI BREAK"(w341) -> ()
        n257 = global write "Robot Global Data.vi" "ACL YAW RST"(w339) -> ()
        n258 = global write "Robot Global Data.vi" "JOY1 H"(w350) -> ()
        n259 = global write "Robot Global Data.vi" "GAT E"(w349) -> ()
        n260 = global write "Robot Global Data.vi" "GAT D"(w348) -> ()
        n261 = global write "Robot Global Data.vi" "BTN A"(w347) -> ()
        n262 = global write "Robot Global Data.vi" "BTN B"(w346) -> ()
        n263 = global write "Robot Global Data.vi" "BTN Y"(w345) -> ()
        n264 = global write "Robot Global Data.vi" "BTN LB"(w344) -> ()
      }
    }
    frame "Your Turn" {
    }
  }
  n265 = disable-structure shown="Disabled" {
    frame Disabled {
      n266 = while {
        shift-right: [w632] -> _
        shift-left: _ -> [w634]
        shift-right: [w630] -> _
        shift-left: _ -> [w631]
        stop <- FALSE stop-if-true
        n267 = global read "Robot Global Data.vi" "DISTANCE ECE(m)"() -> (w627)
        n268 = global read "Robot Global Data.vi" "ACL PITCH"() -> (w628:dbl)
        n269 = global read "Robot Global Data.vi" "CUBE ITK INF"() -> (w625:bool)
        n270 = Wait (ms)(milliseconds to wait=u32 5) -> ()  [unwired: 1 out]
        n271 = case shown="\"ESTABILIZA EQUILIBRIO\"" w634 {
          selector: w634 -> [w644 w656 w665 w699 w709 w729 w738 w752 w764 _ _]
          tunnel: [w645 w654 w666 w700 w708 w730 w739 w753 w764 _ _] -> w632
          tunnel: w631 -> [w642 _ w663 _ w710 _ _ _ _ _ _]
          tunnel: [w643 _ w664 _ w711 _ _ _ _ _ _] -> w630
          tunnel: [TRUE FALSE TRUE FALSE TRUE FALSE FALSE TRUE FALSE _ _] -> _
          tunnel: w627 -> [_ _ _ _ _ _ _ _ _ _ _]
          tunnel: [0.0 "ACELERA敲O 1 A3 2" 0.0 0.0 ("ACELERA敲O 3 A3 2") 0.0 w721 0.2 ("ACELERA敲O 3 A3 2") "ACELERA敲O 3 A3 2" w755 _ _] -> _
          tunnel: w628 -> [_ _ _ _ _ _ w734 w746 _ _ _]
          tunnel: [TRUE TRUE TRUE TRUE TRUE TRUE TRUE TRUE TRUE _ _] -> _
          tunnel: [0.0 0.0 ("ACELERA敲O 3 A3 2") 0.0 w689 0.0 _ _ 0.0 w756 _ _] -> _
          tunnel: [_ _ FALSE w676 FALSE _ _ _ _ _ _] -> _
          tunnel: [_ _ FALSE w675 FALSE _ _ _ _ _ _] -> w626
          tunnel: w625 -> [_ _ _ w674 _ _ _ _ _ _ _]
          frame "INICIO", Default {
            n272 = Divide(x="TIMER 1 A3 2", y=5.0) -> (x/y=w639:dbl)
            n273 = Increment(x=w642) -> (x+1=w643:dbl)
            n274 = Greater Or Equal?(x=w642, y=w639) -> (x >= y?=w647:bool)
            n275 = Select(t=ENUM_01."ANDA PARA FRENTE", s=w647, f=w644) -> (s? t:f=w645:T6)
          }
          frame "ANDA PARA FRENTE" {
            n276 = Greater Or Equal?(y="DISTANCIA A\nPERCORRER 1 A3 2") -> (x >= y?=w655:bool)  [unwired: 1 in]
            n277 = Select(t=ENUM_01."ESPERA 1", s=w655, f=w656) -> (s? t:f=w654:T6)
          }
          frame "ESPERA 1" {
            n278 = Divide(x="TIMER 2 A3 2", y=5.0) -> (x/y=w668:dbl)
            n279 = Increment(x=w663) -> (x+1=w664:dbl)
            n280 = Greater Or Equal?(x=w663, y=w668) -> (x >= y?=w671:bool)
            n281 = Select(t=ENUM_01."ANDA PARA TRAS", s=w671, f=w665) -> (s? t:f=w666:T6)
          }
          frame "ANDA PARA TRAS" {
            n282 = Not(x=w674) -> (.not. x?=w673:bool)
            n283 = Less Or Equal?(y="DISTANCIA A\nPERCORRER 2 A3 2") -> (x <= y?=w696:bool)  [unwired: 1 in]
            n284 = Select(t=ENUM_01."ESPERA 2", s=w696, f=w699) -> (s? t:f=w700:T6)
            n285 = Less Or Equal?(y=-2.0) -> (x <= y?=w672:bool)  [unwired: 1 in]
            n286 = Less Or Equal?(y=-0.1) -> (x <= y?=w684:bool)  [unwired: 1 in]
            n287 = Not(x=w672) -> (.not. x?=w687:bool)
            n288 = Less Or Equal?(y=-0.2) -> (x <= y?=w686:bool)  [unwired: 1 in]
            n289 = Add(x="ACELERA敲O 2 A3 2", y=0.2) -> (x+y=w694:dbl)
            n290 = And(x=w673, y=w684) -> (x .and. y?=w683:bool)
            n291 = Select(t=TRUE, s=w683, f=FALSE) -> (s? t:f=w676:bool)
            n292 = And(x=w687, y=w686) -> (x .and. y?=w685:bool)
            n293 = Select(t=w694, s=w672, f="ACELERA敲O 2 A3 2") -> (s? t:f=w690:dbl)
            n294 = Negate(x=w690) -> (-x=w689:dbl)
            n295 = Select(t=TRUE, s=w685, f=FALSE) -> (s? t:f=w675:bool)
          }
          frame "ESPERA 2" {
            n296 = Divide(x="TIMER 3 A3 2", y=5.0) -> (x/y=w713:dbl)
            n297 = Increment(x=w710) -> (x+1=w711:dbl)
            n298 = Greater Or Equal?(x=w710, y=w713) -> (x >= y?=w704:bool)
            n299 = Select(t=ENUM_01."VOLTA PARA A RAMPA", s=w704, f=w709) -> (s? t:f=w708:T6)
          }
          frame "VOLTA PARA A RAMPA" {
            n300 = Greater Or Equal?(y="DISTANCE\nVOLTAR") -> (x >= y?=w725:bool)  [unwired: 1 in]
            n301 = Divide(x="DISTANCE\nVOLTAR", y=2.0) -> (x/y=w722:dbl)
            n302 = Greater Or Equal?(y=w722) -> (x >= y?=w720:bool)  [unwired: 1 in]
            n303 = Select(t=ENUM_01."INICIO EQUILIBRAR", s=w725, f=w729) -> (s? t:f=w730:T6)
            n304 = Divide(x="ACELERA敲O\n 3 A3 4", y=2.0) -> (x/y=w719:dbl)
            n305 = Select(t=w719, s=w720, f="ACELERA敲O\n 3 A3 4") -> (s? t:f=w721:dbl)
          }
          frame "INICIO EQUILIBRAR" {
            n306 = Less Or Equal?(x=w734, y=-11.0) -> (x <= y?=w732:bool)
            n307 = Select(t=ENUM_01."ESTABILIZA EQUILIBRIO", s=w732, f=w738) -> (s? t:f=w739:T6)
          }
          frame "ESTABILIZA EQUILIBRIO" {
            n308 = Add(x="CONTROL FREIO A3 2", y=1.0) -> (x+y=w744:dbl)
            n309 = Greater Or Equal?(x=w746, y="CONTROL FREIO A3 2") -> (x >= y?=w748:bool)
            n310 = Less Or Equal?(x=w746, y=w744) -> (x <= y?=w747:bool)
            n311 = And(x=w748, y=w747) -> (x .and. y?=w745:bool)
            n312 = Select(t=ENUM_01."FREIO", s=w745, f=w752) -> (s? t:f=w753:T6)
          }
          frame "FREIO" {
            w759 = 0.0 ("y")
            # "0,5"
            n313 = Negate() -> (-x=w754:dbl)  [unwired: 1 in]
            n314 = call-poly <vilib>:"PID.vi"("output range"=cluster{"output high":dbl, "output low":dbl} {"output high"=-0.5, "output low"=0.5}, "PID gains"=T5 {"proportional gain (Kc)"=25.0, "integral time (Ti, min)"=0.0, "derivative time (Td, min)"=0.0}, "process variable"=w754, "setpoint"=0.0) -> ("output"=w757:dbl)  [unwired: 6 in, 1 out]
            n315 = Greater?(x=w757, y=w759) -> (0:w761:bool)
            n316 = Less?(x=w757, y=w759) -> (x < y?=w760:bool)
            n317 = Select(t=w757, s=w760, f=w759) -> (s? t:f=w758:dbl)
            n318 = Select(t=w757, s=w761, f=w759) -> (s? t:f=w756:dbl)
            n319 = Negate(x=w758) -> (-x=w755:dbl)
          }
          frame "ESPERA 3" {
          }
          frame "EQUILIBRIO" {
          }
        }
        n320 = global write "Robot Global Data.vi" "CUBE ITK INF"(w626) -> ()
        n321 = global read "Robot Global Data.vi" "BTN1"() -> ()  [unwired: 1 in]
        n322 = global read "Robot Global Data.vi" "RST ECE"() -> ()  [unwired: 1 in]
        n323 = global read "Robot Global Data.vi" "FREIO EN"() -> ()  [unwired: 1 in]
        n324 = global read "Robot Global Data.vi" "AXES3"() -> ()  [unwired: 1 in]
        n325 = global read "Robot Global Data.vi" "AXES2"() -> ()  [unwired: 1 in]
      }
    }
    frame Enabled {
    }
  }
